vi "Send Graphite Metrics.vi"(8 "error in (no error)":errorcluster, 10 "Metriics":cluster{"metric":string, "value":dbl}[](array[cluster]), 11 "TCP Network Connection in":refnum<k5>) -> (0 "error out":errorcluster, 2 "Messages":string[](array[string]), 3 "TCP Network Connection out":refnum<k5>)   [LabVIEW 2023]
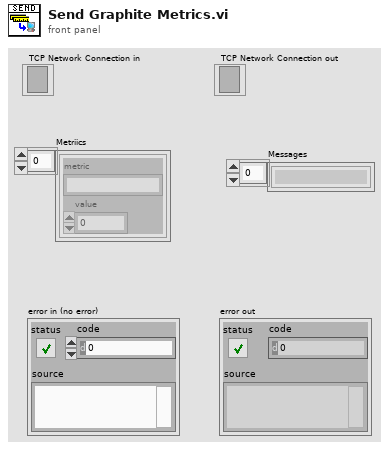
[diagram p1: front panel]
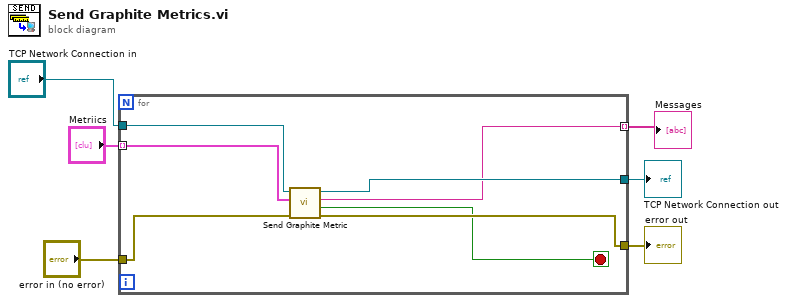
[diagram p0: block diagram]
diagram:
  n1 = for {
    tunnel: "Metriics" -> [w9] mode=indexing
    tunnel: "TCP Network Connection in" -> [w13]
    tunnel: "error in (no error)" -> [w12]
    tunnel: [w11] -> w4
    tunnel: [w10] -> w5
    tunnel: [w7] -> w1 mode=indexing
    stop <- w8 stop-if-true
    n2 = call "Send Graphite Metric.vi"("error in (no error)"=w12, "Cluster"=w9, "TCP Network Connection in"=w13) -> ("error out"=w10:errorcluster, "status"=w8:bool, "Message"=w7:string, "TCP Network Connection out"=w11:refnum<k5>)  [unwired: 5 in]
  }
  "error out" <- w5
  "TCP Network Connection out" <- w4
  "Messages" <- w1
